vi "Mean Instantaneous Frequency or Bandwidth (MIF or MIB).vi"() -> ()   [LabVIEW 2023]
doc: "This example shows how to compute the mean instantaneous frequency (MIF) and the mean instantaneous bandwidth (MIB) by using the TFA Mean Instantaneous Frequency VI and TFA Mean Instantaneous Bandwidth VI, respectively. When a signal is contaminated by heavy noise, the MIF and the MIB estimated from the spectrogram may include errors. You can specify different values for <B>Trimmed Percent</B> to improve the estimation precision.\n\n<b>Instructions:</b>\n1) Run this VI.\n2) Observe the MIF and MIB of the Doppler signal.\n3) Browse the Block Diagram of this example to learn how to compute the MIF and MIB by using the Time Frequency Analysis Tools."
uses:
  <vilib>/addons/Time Frequency Analysis/typedefs.llb/TFA Data.ctl
  <vilib>/addons/Time Frequency Analysis/Spectrogram.llb/TFA STFT Spectrogram (Complex).vi
  <vilib>/addons/Time Frequency Analysis/_control.llb/TFA Configure Spectrogram Indicator (Predefined Color Table).vi
  <vilib>/addons/_Advanced Signal Processing/NI_AdvSigProcTFA.lvlib
  <vilib>/Analysis/NI_AALBase.lvlib
panel:
  out "aspt-left-top":bool
  in  "Trimmed percent":cluster{"upper":dbl, "lower":dbl}={"upper"=0.0, "lower"=40.0} {"lower" min=0.0 max=100.0 format="%#_g %"; "upper" min=0.0 max=100.0 format="%#_g %"}
  out "Doppler Signal":waveform(dbl)[](graph)
  in  "Frequency bins":i32=512
  in  "Time steps":i32=4
  out "Mean Instantaneous Bandwidth":cluster{"t0":dbl, "dt":dbl, "bandwidth":dbl[]}(graph)
  out "Mean Instantaneous Frequency":cluster{"t0":dbl, "dt":dbl, "frequency":dbl[]}(graph)
  out "Spectrogram":dbl[][](graph)
  # "Overview: Shows how to compute the mean instantaneous frequency (MIF) and the mean instantaneous bandwidth (MIB) by using the TFA Mean Instantaneous Frequency VI and TFA Mean Instantaneous Bandwidth VI, respectively. \nRequirements: LabVIEW Full Development System, Advanced Signal Processing Toolkit\nInstructions: \n1. Run this VI.\n2. Observe the MIF and MIB of the Doppler signal.\n3. Browse the block diagram of this example to learn how to compute the MIF and MIB by using the Time Frequency Analysis Tools."
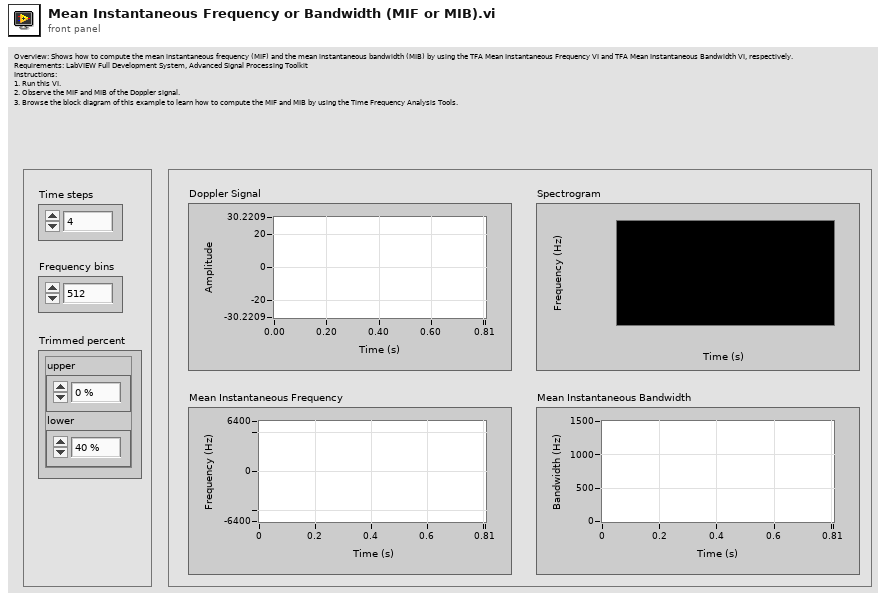
[diagram p1: front panel]
types:
  T1 = typedef "NI_AdvSigProcTFA.lvlib/TFA Data.ctl" = u16
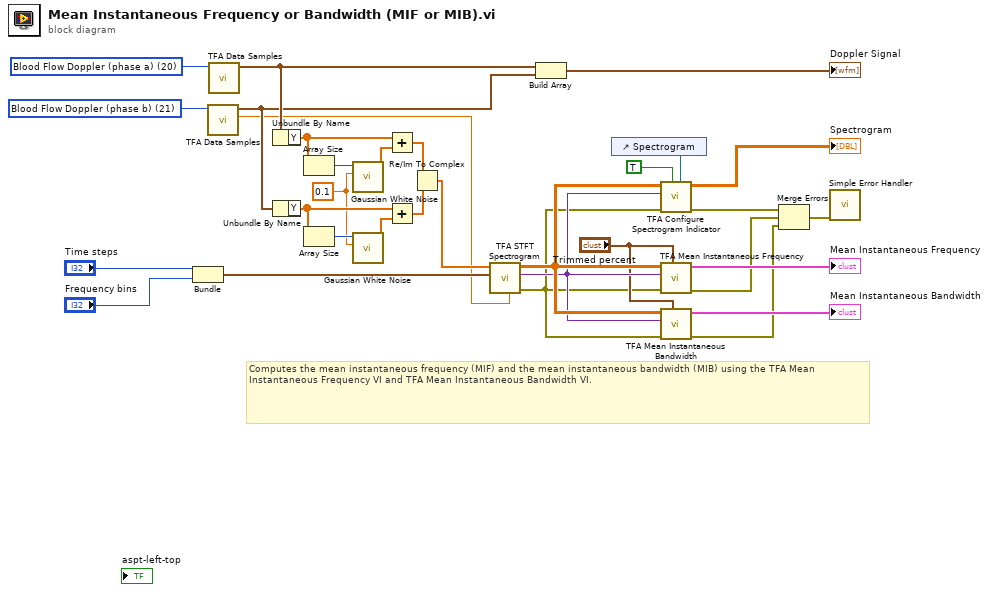
[diagram p0: block diagram]
diagram:
  w6 = T1 21 items=["PC Fan"=0, "Noisy Chirps"=1, "TDR 1"=2, "TDR 2"=3, "Liquefaction"=4, "Liquefaction Free"=5, "Aneurysm"=6, "Bat"=7, "RF"=8, "Two Gaussian"=9, "Three Gaussian"=10, "Chirp"=11, "Gaussian Chirp"=12, "Cross Chirp"=13, "Doppler"=14, "HOP"=15, "TF Sine"=16, "Three Tone"=17, "Four Tone"=23, "Blood Flow Doppler (phase a)"=20, "Blood Flow Doppler (phase b)"=21, "Heart sound"=22, "-"=18, "Random Noise"=19] ("data")
  w7 = T1 20 items=["PC Fan"=0, "Noisy Chirps"=1, "TDR 1"=2, "TDR 2"=3, "Liquefaction"=4, "Liquefaction Free"=5, "Aneurysm"=6, "Bat"=7, "RF"=8, "Two Gaussian"=9, "Three Gaussian"=10, "Chirp"=11, "Gaussian Chirp"=12, "Cross Chirp"=13, "Doppler"=14, "HOP"=15, "TF Sine"=16, "Three Tone"=17, "Four Tone"=23, "Blood Flow Doppler (phase a)"=20, "Blood Flow Doppler (phase b)"=21, "Heart sound"=22, "-"=18, "Random Noise"=19] ("data")
  w8 = 0.1 ("standard deviation")
  # "Computes the mean instantaneous frequency (MIF) and the mean instantaneous bandwidth (MIB) using the TFA Mean Instantaneous Frequency VI and TFA Mean Instantaneous Bandwidth VI."
  n1 = Bundle("Time steps"="Time steps", "Frequency bins"="Frequency bins") -> (w29:cluster{"Time steps":i32, "Frequency bins":i32})  [unwired: 1 out]
  n2 = call <vilib>:"TFA Data Samples.vi"("data"=w6) -> ("sampling rate"=w18:dbl, "signal"=w19:waveform(dbl))  [unwired: 9 out]
  n3 = call <vilib>:"TFA Data Samples.vi"("data"=w7) -> ("signal"=w20:waveform(dbl))  [unwired: 10 out]
  n4 = Unbundle By Name(w20) -> ("Y"=w14:dbl[])
  n5 = Unbundle By Name(w19) -> ("Y"=w10:dbl[])
  n6 = Array Size(array=w14) -> (size(s)=w16:i32)
  n7 = Array Size(array=w10) -> (size(s)=w11:i32)
  n8 = call <vilib>:"Gaussian White Noise.vi"("standard deviation"=w8, "samples"=w16) -> ("Gaussian noise pattern"=w13:dbl[])  [unwired: 8 in, 1 out]
  n9 = call <vilib>:"Gaussian White Noise.vi"("standard deviation"=w8, "samples"=w11) -> ("Gaussian noise pattern"=w12:dbl[])  [unwired: 8 in, 1 out]
  n10 = Add(x=w14, y=w13) -> (x+y=w15:dbl[])
  n11 = Add(x=w10, y=w12) -> (x+y=w9:dbl[])
  n12 = Re/Im To Complex(1:w9, 2:w15) -> (0:w22:cdb[])
  n13 = call-poly <vilib>:"TFA STFT Spectrogram.vi"("sampling rate"=w18, "time-frequency sampling info"=w29, "signal"=w22) -> ("error out"=w5:errorcluster, "scale info"=w27:variant, "spectrogram"=w28:dbl[][])  [unwired: 2 in, 4 out]
  n14 = Build Array(w20, w19) -> (→"Doppler Signal":waveform(dbl)[])
  n15 = control-ref of="Spectrogram"() -> (w26:refnum<vi>)
  n16 = call-poly <vilib>:"TFA Configure Spectrogram Indicator.vi"("reference of TF spectrogram indicator"=w26, "dB on? (F)"=TRUE ("dB? (F)"), "error in (no error)"=w5, "scale info"=w27, "spectrogram"=w28) -> ("error out"=w4:errorcluster, "TF spectrogram indicator"=→"Spectrogram":dbl[][])  [unwired: 2 in, 3 out]
  n17 = call <vilib>:"TFA Mean Instantaneous Frequency.vi"("trimmed percent"="Trimmed percent", "error in (no error)"=w5, "scale info"=w27, "spectrogram"=w28) -> ("error out"=w3:errorcluster, "MIF"=→"Mean Instantaneous Frequency":cluster{"t0":dbl, "dt":dbl, "frequency":dbl[]})  [unwired: 6 out]
  n18 = call <vilib>:"TFA Mean Instantaneous Bandwidth.vi"("trimmed percent"="Trimmed percent", "error in (no error)"=w5, "scale info"=w27, "spectrogram"=w28) -> ("error out"=w1:errorcluster, "MIB"=→"Mean Instantaneous Bandwidth":cluster{"t0":dbl, "dt":dbl, "bandwidth":dbl[]})  [unwired: 6 out]
  n19 = Merge Errors(w4, w3, w1) -> (w2:errorcluster)
  n20 = call <vilib>:"Simple Error Handler.vi"("error in (no error)"=w2) -> ()  [unwired: 4 in, 5 out]
